vi "Constructor-Port.vi"(8 "error in (no error)":errorcluster, 11 "ListenerPort":i32) -> (0 "error out":errorcluster, 3 "ServiceManager out":refnum<class "ServiceManager.lvclass">)   [LabVIEW 2020, in "ServiceManager.lvlib" / "ServiceManager.lvclass"]
uses:
  ServiceManager.lvclass
  ServiceManager.lvclass/ServiceManager.ctl
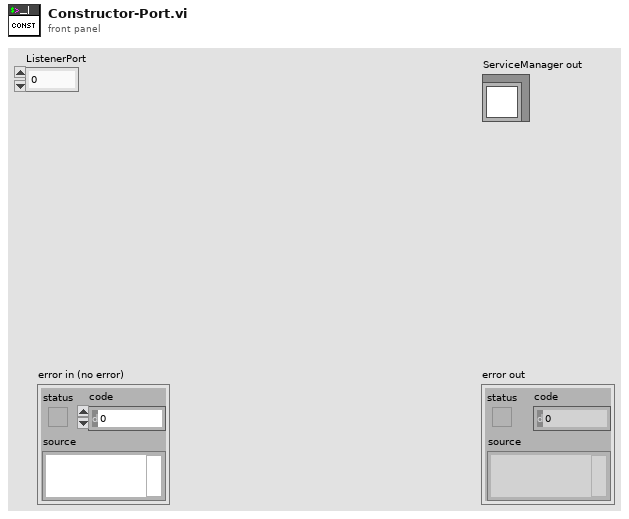
[diagram p1: front panel]
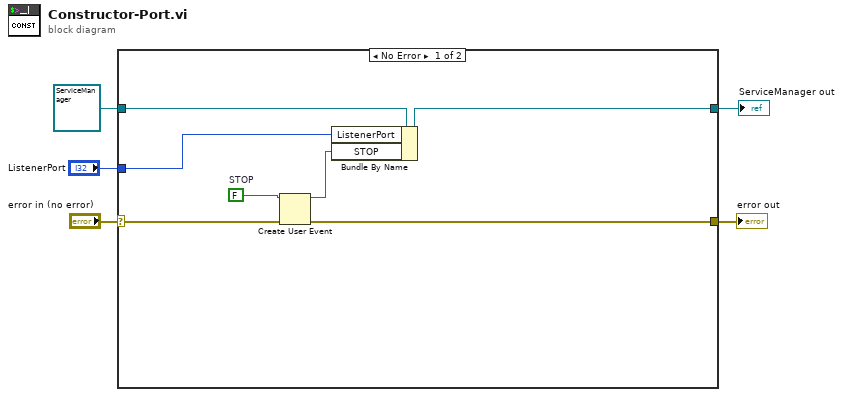
[diagram p0: block diagram]
diagram:
  n1 = case shown="No Error" "error in (no error)" {
    selector: "error in (no error)" -> [w9 w14]
    tunnel: [w8 w14] -> w4
    tunnel: [w11 w13] -> w2
    tunnel: refnum<class "ServiceManager.lvclass"> refnum ("ServiceManager in") -> [w12 w13]
    tunnel: "ListenerPort" -> [w10 _]
    frame No Error {
      w7 = FALSE  # STOP
      n2 = Create User Event(user event datatype=w7, error in=w9) -> (user event=w6:refnum<user-event>, error out=w8:errorcluster)
      n3 = Bundle By Name(cluster=w12, "ListenerPort"=w10, "STOP"=w6) -> (w11:refnum<class "ServiceManager.lvclass">)
    }
    frame Error {
    }
  }
  "error out" <- w4
  "ServiceManager out" <- w2
